vi "Impedance_Analyzer_Main.vi"() -> ()   [LabVIEW 2022 SP3]
uses:
  <vilib>/Math Plots/2D Math Plots/2D Compass/2D Compass XCtrl/2D Compass.xctl
  <vilib>/Math Plots/2D Math Plots/2D Compass/2D Compass Datatype/2D Compass Datatype.lvclass
  <vilib>/Analysis/1siggen.llb/Ramp Pattern by Samples.vi
  <vilib>/Analysis/baseanly.llb/Mean (DBL).vi
  <vilib>/Math Plots/2D Math Plots/2D Compass/2D Compass Datatype/Public/Plot Helper (Vector).vi
  <vilib>/Analysis/NI_AALBase.lvlib
panel:
  in  "Shunt Gain Setting 3":bool
  in  "ResetLine-Shunt 2":tag="PXI1Slot2/port0/line3"
  in  "SetLine-Shunt 2":tag="PXI1Slot2/port0/line2"
  in  "SetLine-Shunt":tag="PXI1Slot2/port0/line0"
  in  "ResetLine-Shunt":tag="PXI1Slot2/port0/line1"
  in  "Shunt Gain Setting":bool
  out "Test Number 3":i32=2
  in  "Saving Cluster":T1={"Experiment Title"="Experiment Title", "Save Path"=path "C:/Users/MPI/Downloads", "File Name String"="TestStats", "Meta-Data Array"=[]}
  out "Main loop has stopped":bool
  out "Duration of last non-idle state (sec)":dbl format="%.3g"
  out "Start of current operation":timestamp=timestamp(3746717327.8850594 s since 1904-01-01)
  out "Current system state":string="Idle"
  in  "stop":bool
  in  "Tab Control":T2(tab)
  in  "Test Params Cluster":T3={"Test Freq. (Hz)"=100.0, "Output Signal Amplitude\nVolts Pk"=0.6, "Sampling Time (s)"=0.1, "Sampling Rate (Hz)"=1000000.0, "Output Channel"="PXI1Slot2/ao0", "Current Channel"="PXI1Slot2/ai0", "Voltage Channel"="PXI1Slot2/ai1", "Trigger Channel"="/PXI1Slot2/ao/StartTrigger", "Number of runs"=5} {"Sampling Rate (Hz)" format="%#_6p"}
  in  "LCR Params":T4={"Rg_Vmon"=10000.0, "Rg_Imon"=10000.0, "ESL_Cal"=3.9470118585717184e-07, "ESR_Cal"=-0.006312489258536832, "Cp_Cal"=0.0, "Rp_Cal"=1000000000.0, "UseCorrection"=TRUE, "R_Shunt"=100.0, "RLoad"=1000000000.0, "RLoad_Meas"=1000000000.0} {"RLoad_Meas" format="%#_6p"; "RLoad" format="%#_6p"; "R_Shunt" format="%#_6p"; "Rg_Vmon" format="%#_6p"; "Rg_Imon" format="%#_6p"; "ESL_Cal" format="%#_6p"; "ESR_Cal" format="%#_6p"; "Cp_Cal" format="%#_6p"; "Rp_Cal" format="%#_6p"}
  out "mean Real(Z)":dbl=-0.006312489258536832
  in  "Open Comp":bool
  in  "Short Comp":bool
  in  "Number of Tests\n-Compensation":i32=10 format="%#.6p"
  in  "Save final stats - Compensation":bool
  out "Histogram Graph Phase 2":T5(graph)={"X Values"=[0.059615962899507886, 0.05963710991927518, 0.05965825693904247, 0.05967940395880976, 0.05970055097857705, 0.05972169799834434, 0.05974284501811163, 0.059763992037878924, 0.059785139057646215, 0.059806286077413506], "Histogram: h(x)"=[1, 0, 0, 0, 0, 0, 0, 0, 0, 1]}
  out "Histogram Graph Phase 3":T5(graph)={"X Values"=[95.20701436407293, 95.2415389303248, 95.27606349657665, 95.31058806282851, 95.34511262908038, 95.37963719533224, 95.4141617615841, 95.44868632783596, 95.48321089408782, 95.51773546033968], "Histogram: h(x)"=[1, 0, 0, 2, 1, 1, 2, 1, 1, 1]}
  out "Histogram Graph Mag 3":T5(graph)={"X Values"=[0.05657083132191394, 0.05658175212173795, 0.05659267292156196, 0.05660359372138597, 0.05661451452120998, 0.05662543532103399, 0.056636356120858, 0.05664727692068201, 0.05665819772050602, 0.056669118520330033], "Histogram: h(x)"=[1, 0, 1, 0, 1, 0, 4, 1, 1, 1]}
  out "Histogram Graph Mag 2":T5(graph)={"X Values"=[91.42562370503113, 92.47253112610193, 93.51943854717271, 94.5663459682435, 95.61325338931428, 96.66016081038507, 97.70706823145585, 98.75397565252663, 99.80088307359742, 100.8477904946682], "Histogram: h(x)"=[1, 0, 0, 0, 0, 0, 0, 0, 0, 1]}
  out "Open Comp Output":T6 {"Mean |Z|" format="%#_6p"; "standard deviation |Z|" format="%#_6p"; "Mean Phase" format="%#_6p"; "standard deviation Phase" format="%#_6p"; "mean Ls" format="%#_6p"; "Standard dev. Ls" format="%#_6p"; "mean Real(Z)" format="%#_6p"; "Std. dev Real(Z)" format="%#_6p"; "mean Cs" format="%#_6p"; "Std. Dev. Cs" format="%#_6p"; "Mean Rp" format="%#_6p"; "Std. Dev. Rp" format="%#_6p"; "Mean Cp" format="%#_6p"; "Std. Dev. Cp" format="%#_6p"}
  out "Short Comp Output":T6={"Mean |Z|"=0.05952615930946873, "standard deviation |Z|"=0.00033736666024453306, "Mean Phase"=96.11062136035359, "standard deviation Phase"=5.234732094839484, "mean Ls"=3.9470118585717184e-07, "Standard dev. Ls"=4.734939240935585e-09, "mean Real(Z)"=-0.006312489258536832, "Std. dev Real(Z)"=0.005405474422231036, "mean Cs"=-0.00011330769248196087, "Std. Dev. Cs"=1.3530545947492297e-06, "Mean Rp"=-1.5539543323796643, "Std. Dev. Rp"=1.9485966785903661, "Mean Cp"=-0.00011139347112511099, "Std. Dev. Cp"=1.2568699443711718e-06} {"Mean |Z|" format="%#_6p"; "standard deviation |Z|" format="%#_6p"; "Mean Phase" format="%#_6p"; "standard deviation Phase" format="%#_6p"; "mean Ls" format="%#_6p"; "Standard dev. Ls" format="%#_6p"; "mean Real(Z)" format="%#_6p"; "Std. dev Real(Z)" format="%#_6p"; "mean Cs" format="%#_6p"; "Std. Dev. Cs" format="%#_6p"; "Mean Rp" format="%#_6p"; "Std. Dev. Rp" format="%#_6p"; "Mean Cp" format="%#_6p"; "Std. Dev. Cp" format="%#_6p"}
  out "Ls Chart 3":dbl(graph)
  out "ESR 3":dbl(graph)
  out "Ls Chart 2":dbl(graph)=3.933790349340922e-07
  out "ESR Short":dbl(graph)=-0.00624352369104645
  out "Current Short Comp. Results":T7={"|Z|"=0.05915622895148479, "Phase(Z)"=96.05844988136137, "Re(Z)"=-0.00624352369104645, "Imag(Z)"=0.058825826264318884, "Ls"=3.933790349340922e-07, "Cs"=-0.00011367766349435693, "Rp"=-0.5604942972794196, "Cp"=-0.00011241137195737807} {"|Z|" format="%#_6p"; "Phase(Z)" format="%#_6p"; "Re(Z)" format="%#_6p"; "Imag(Z)" format="%#_6p"; "Ls" format="%#_6p"; "Cs" format="%#_6p"; "Rp" format="%#_6p"; "Cp" format="%#_6p"}
  out "Current Open Comp. Results":T7={"|Z|"=0.05656537092200194, "Phase(Z)"=95.45920483054104, "Re(Z)"=-0.005381459479146001, "Imag(Z)"=0.056308801100875626, "Ls"=3.584729613913086e-07, "Cs"=-0.00011305866221997783, "Rp"=-0.5945675517845621, "Cp"=-0.00011203536283595137} {"|Z|" format="%#_6p"; "Phase(Z)" format="%#_6p"; "Re(Z)" format="%#_6p"; "Imag(Z)" format="%#_6p"; "Ls" format="%#_6p"; "Cs" format="%#_6p"; "Rp" format="%#_6p"; "Cp" format="%#_6p"}
  in  "Update Variables":bool
  out "Progress 3":i32(slide)=66 scale=0.0..100.0
  in  "Samples\nShort Comp":i32=3 format="%#.6p"
  out "Debug Cluster-Short":T8={"detected fundamental frequency"=23800.1359424882, "THD-IMon"=0.04051349221415451, "THD-VMon"=0.0, "IMon-Ampl"=0.9038077003743037, "VMon-Ampl"=0.0007818146474553097} {"VMon-Ampl" format="%.2p"; "IMon-Ampl" format="%.2p"; "THD-VMon" format="%.2p"; "THD-IMon" format="%.2p"; "detected fundamental frequency" format="%.2p"}
  out "Debug Cluster-Open":T8 {"VMon-Ampl" format="%.2p"; "IMon-Ampl" format="%.2p"; "THD-VMon" format="%.2p"; "THD-IMon" format="%.2p"; "detected fundamental frequency" format="%.2p"}
  in  "Start Stats":bool
  in  "Save final stats":bool
  out "Histogram Graph Phase":T5(graph)={"X Values"=[100.0, 100.0, 100.0, 100.0, 100.0, 100.0, 100.0, 100.0, 100.0, 100.0], "Histogram: h(x)"=[0, 0, 0, 0, 0, 0, 0, 0, 0, 2]}
  out "Progress":i32(slide)=66 scale=0.0..100.0
  out "Inductance Chart":dbl(graph)=3.606768335066755e-19
  out "output cluster":T6={"Mean |Z|"=100.0, "standard deviation |Z|"=0.0, "Mean Phase"=179.99999999999997, "standard deviation Phase"=0.0, "mean Ls"=3.606768335066755e-19, "Standard dev. Ls"=0.0, "mean Real(Z)"=-100.0, "Std. dev Real(Z)"=0.0, "mean Cs"=-112367830.95520051, "Std. Dev. Cs"=1.8250120749944284e-08, "Mean Rp"=-100.0, "Std. Dev. Rp"=0.0, "Mean Cp"=-3.6067683350667554e-23, "Std. Dev. Cp"=0.0} {"Mean |Z|" format="%#_6p"; "standard deviation |Z|" format="%#_6p"; "Mean Phase" format="%#_6p"; "standard deviation Phase" format="%#_6p"; "mean Ls" format="%#_6p"; "Standard dev. Ls" format="%#_6p"; "mean Real(Z)" format="%#_6p"; "Std. dev Real(Z)" format="%#_6p"; "mean Cs" format="%#_6p"; "Std. Dev. Cs" format="%#_6p"; "Mean Rp" format="%#_6p"; "Std. Dev. Rp" format="%#_6p"; "Mean Cp" format="%#_6p"; "Std. Dev. Cp" format="%#_6p"}
  out "Current Run Results":T7={"|Z|"=100.0, "Phase(Z)"=179.99999999999997, "Re(Z)"=-100.0, "Imag(Z)"=5.6654984523230034e-14, "Ls"=3.606768335066755e-19, "Cs"=-112367830.95520052, "Rp"=-100.0, "Cp"=-3.6067683350667554e-23} {"|Z|" format="%#_6p"; "Phase(Z)" format="%#_6p"; "Re(Z)" format="%#_6p"; "Imag(Z)" format="%#_6p"; "Ls" format="%#_6p"; "Cs" format="%#_6p"; "Rp" format="%#_6p"; "Cp" format="%#_6p"}
  out "Capacitance Chart":dbl(graph)=-112367830.95520052
  out "Phase Chart":dbl(graph)=179.99999999999997
  out "Real(Z) Chart":dbl(graph)=-100.0
  out "|Z| over time":dbl(graph)=100.0
  out "Test Number":i32=2
  in  "samples":i32=3 format="%#.6p"
  in  "Save Every\nRun File?":bool
  out "Debug Cluster-Stats":T8 {"VMon-Ampl" format="%.2p"; "IMon-Ampl" format="%.2p"; "THD-VMon" format="%.2p"; "THD-IMon" format="%.2p"; "detected fundamental frequency" format="%.2p"}
  in  "Start Freq. Sweep":bool
  in  "Save sweep":bool
  out "Mag Phase Graph":cluster{dbl[], dbl[]}[](graph)=[{[15000.0, 15213.695804509916, 15430.43600214417, 15650.263964505297, 15873.22368108446, 16099.359768064103, 16328.717477246168, 16561.34270510718, 16797.28200198266, 17036.582581382234, 17279.292329437434, 17525.459814484173, 17775.134296781664, 18028.365738369826, 18285.204813067154, 18545.70291661091, 18809.91217694204, 19077.8854646362, 19349.67640348376, 19625.339381220358, 19904.929560410354, 20188.502889485353, 20476.11611393997, 20767.82678768709, 21063.69328457491, 21363.774810068015, 21668.13141309509, 21976.823998064945, 22289.914337054226, 22607.46508216848, 22929.539778079397, 23256.202874740644, 23587.519740284875, 23923.556674104446, 24264.38092011853, 24610.060680229126, 24960.665127969078, 25316.264422344004, 25676.9297218719, 26042.73319882256, 26413.748053659852, 26790.048529689782, 27171.709927917225, 27558.80862211431, 27951.42207410347, 28349.628849258188, 28753.50863222483, 29163.142242867896, 29578.611652443007, 30000.0], [99.99999999999999, 100.00000000000001, 100.0, 100.0, 100.00000000000001, 100.00000000000001, 100.0, 100.0, 100.0, 99.99999999999999, 100.0, 100.0, 99.99999999999999, 100.00000000000001, 100.0, 100.0, 99.99999999999999, 100.0, 100.00000000000001, 100.00000000000001, 100.00000000000001, 99.99999999999999, 100.0, 99.99999999999999, 100.00000000000001, 100.00000000000001, 100.00000000000001, 100.00000000000001, 100.0, 99.99999999999999, 99.99999999999997, 100.0, 100.0, 99.99999999999999, 100.0, 99.99999999999999, 100.0, 100.00000000000001, 99.99999999999999, 100.0, 100.0, 100.00000000000001, 100.0, 100.0, 100.00000000000001, 100.00000000000001, 100.0, 100.0, 100.0, 100.00000000000001]}, {[15000.0, 15213.695804509916, 15430.43600214417, 15650.263964505297, 15873.22368108446, 16099.359768064103, 16328.717477246168, 16561.34270510718, 16797.28200198266, 17036.582581382234, 17279.292329437434, 17525.459814484173, 17775.134296781664, 18028.365738369826, 18285.204813067154, 18545.70291661091, 18809.91217694204, 19077.8854646362, 19349.67640348376, 19625.339381220358, 19904.929560410354, 20188.502889485353, 20476.11611393997, 20767.82678768709, 21063.69328457491, 21363.774810068015, 21668.13141309509, 21976.823998064945, 22289.914337054226, 22607.46508216848, 22929.539778079397, 23256.202874740644, 23587.519740284875, 23923.556674104446, 24264.38092011853, 24610.060680229126, 24960.665127969078, 25316.264422344004, 25676.9297218719, 26042.73319882256, 26413.748053659852, 26790.048529689782, 27171.709927917225, 27558.80862211431, 27951.42207410347, 28349.628849258188, 28753.50863222483, 29163.142242867896, 29578.611652443007, 30000.0], [-180.0, -180.0, -180.0, -180.0, -179.99999999999997, -180.0, -180.0, 179.99999999999997, -180.0, -180.0, -179.99999999999997, -179.99999999999997, 180.0, 179.99999999999994, 180.0, -180.0, -180.0, -180.0, -180.0, -179.99999999999997, 180.0, -179.99999999999997, -180.0, 180.0, 179.99999999999997, 179.99999999999997, 180.0, 180.0, 179.99999999999997, 180.0, -180.0, -180.0, 180.0, -180.0, 180.0, 179.99999999999997, 180.0, 180.0, 179.99999999999997, 180.0, 180.0, 179.99999999999997, 179.99999999999997, -180.0, -180.0, 180.0, 180.0, -179.99999999999997, -180.0, -180.0]}]
  in  "Freq Sweep Info":T9={"type"=1, "Number of\nTest Freqs"=50, "Start Freq"=15000.0, "Stop Freq"=30000.0} {"Stop Freq" format="%#.4p"; "Start Freq" format="%#.4p"; "type" items=["Linear", "Logarithmic"]}
  out "Current Run Cluster Sweep":T3={"Test Freq. (Hz)"=30000.0, "Output Signal Amplitude\nVolts Pk"=0.1, "Sampling Time (s)"=0.001, "Sampling Rate (Hz)"=2000000.0, "Output Channel"="SimDev1/ao0", "Current Channel"="SimDev1/ai0", "Voltage Channel"="SimDev1/ai1", "Trigger Channel"="/SimDev1/ao/StartTrigger", "Number of runs"=3}
  out "Current Run Impedances":T7={"|Z|"=100.00000000000001, "Phase(Z)"=-180.0, "Re(Z)"=-100.00000000000001, "Imag(Z)"=-1.2246063538223774e-14, "Ls"=-6.496738485085797e-20, "Cs"=433213885.68422616, "Rp"=-100.00000000000001, "Cp"=6.496738485085795e-24} {"|Z|" format="%#_6p"; "Phase(Z)" format="%#_6p"; "Re(Z)" format="%#_6p"; "Imag(Z)" format="%#_6p"; "Ls" format="%#_6p"; "Cs" format="%#_6p"; "Rp" format="%#_6p"; "Cp" format="%#_6p"}
  out "RealImag Graph":cluster{dbl[], dbl[]}[](graph)=[{[15000.0, 15213.695804509916, 15430.43600214417, 15650.263964505297, 15873.22368108446, 16099.359768064103, 16328.717477246168, 16561.34270510718, 16797.28200198266, 17036.582581382234, 17279.292329437434, 17525.459814484173, 17775.134296781664, 18028.365738369826, 18285.204813067154, 18545.70291661091, 18809.91217694204, 19077.8854646362, 19349.67640348376, 19625.339381220358, 19904.929560410354, 20188.502889485353, 20476.11611393997, 20767.82678768709, 21063.69328457491, 21363.774810068015, 21668.13141309509, 21976.823998064945, 22289.914337054226, 22607.46508216848, 22929.539778079397, 23256.202874740644, 23587.519740284875, 23923.556674104446, 24264.38092011853, 24610.060680229126, 24960.665127969078, 25316.264422344004, 25676.9297218719, 26042.73319882256, 26413.748053659852, 26790.048529689782, 27171.709927917225, 27558.80862211431, 27951.42207410347, 28349.628849258188, 28753.50863222483, 29163.142242867896, 29578.611652443007, 30000.0], [-99.99999999999999, -100.00000000000001, -100.0, -100.0, -100.00000000000001, -100.00000000000001, -100.0, -100.0, -100.0, -99.99999999999999, -100.0, -100.0, -99.99999999999999, -100.00000000000001, -100.0, -100.0, -99.99999999999999, -100.0, -100.00000000000001, -100.00000000000001, -100.00000000000001, -99.99999999999999, -100.0, -99.99999999999999, -100.00000000000001, -100.00000000000001, -100.00000000000001, -100.00000000000001, -100.0, -99.99999999999999, -99.99999999999997, -100.0, -100.0, -99.99999999999999, -100.0, -99.99999999999999, -100.0, -100.00000000000001, -99.99999999999999, -100.0, -100.0, -100.00000000000001, -100.0, -100.0, -100.00000000000001, -100.00000000000001, -100.0, -100.0, -100.0, -100.00000000000001]}, {[15000.0, 15213.695804509916, 15430.43600214417, 15650.263964505297, 15873.22368108446, 16099.359768064103, 16328.717477246168, 16561.34270510718, 16797.28200198266, 17036.582581382234, 17279.292329437434, 17525.459814484173, 17775.134296781664, 18028.365738369826, 18285.204813067154, 18545.70291661091, 18809.91217694204, 19077.8854646362, 19349.67640348376, 19625.339381220358, 19904.929560410354, 20188.502889485353, 20476.11611393997, 20767.82678768709, 21063.69328457491, 21363.774810068015, 21668.13141309509, 21976.823998064945, 22289.914337054226, 22607.46508216848, 22929.539778079397, 23256.202874740644, 23587.519740284875, 23923.556674104446, 24264.38092011853, 24610.060680229126, 24960.665127969078, 25316.264422344004, 25676.9297218719, 26042.73319882256, 26413.748053659852, 26790.048529689782, 27171.709927917225, 27558.80862211431, 27951.42207410347, 28349.628849258188, 28753.50863222483, 29163.142242867896, 29578.611652443007, 30000.0], [1.2246063538223771e-14, 1.2246063538223774e-14, 1.2246063538223773e-14, 1.2246063538223773e-14, 5.665498452323004e-14, 1.2246063538223774e-14, 1.2246063538223773e-14, 5.6654984523230034e-14, 1.2246063538223773e-14, 1.2246063538223771e-14, 5.6654984523230034e-14, 5.6654984523230034e-14, 1.2246063538223771e-14, 1.0106390550823631e-13, 1.2246063538223773e-14, 1.2246063538223773e-14, 1.2246063538223771e-14, 1.2246063538223773e-14, 1.2246063538223774e-14, 5.665498452323004e-14, 1.2246063538223774e-14, 5.665498452323003e-14, 1.2246063538223773e-14, 1.2246063538223771e-14, 5.665498452323004e-14, 5.665498452323004e-14, 1.2246063538223774e-14, 1.2246063538223774e-14, 5.6654984523230034e-14, 1.2246063538223771e-14, 1.224606353822377e-14, 1.2246063538223773e-14, 1.2246063538223773e-14, 1.2246063538223771e-14, 1.2246063538223773e-14, 5.665498452323003e-14, 1.2246063538223773e-14, 1.2246063538223774e-14, 5.665498452323003e-14, 1.2246063538223773e-14, 1.2246063538223773e-14, 5.665498452323004e-14, 5.6654984523230034e-14, 1.2246063538223773e-14, 1.2246063538223774e-14, 1.2246063538223774e-14, 1.2246063538223773e-14, 5.6654984523230034e-14, 1.2246063538223773e-14, 1.2246063538223774e-14]}]
  out "Mean Mag":dbl=100.0 format="%.4p"
  out "Mean Phase":dbl=-7.2 format="%0.2f"
  out "Progress 2":i32(slide)=98 scale=0.0..100.0
  out "Test Number 2":i32=49
  out "Impedance Vector":refnum<class "2D Plot Datatype.lvclass">[](xcontrol) caption="2D Compass"
  out "Progress Single Run":i32(slide)=66 scale=0.0..100.0
  in  "Start Single Meas":bool
  in  "Save Single Impedance":bool
  out "Mean Signal\nImpedance cluster":T7={"|Z|"=0.007576457903951982, "Phase(Z)"=5.046854007613568, "Re(Z)"=0.0075470846798780635, "Imag(Z)"=0.0006665037172486679, "Ls"=4.457031982741531e-09, "Cs"=-0.01003322608680636, "Rp"=0.007605945448499181, "Cp"=-7.764496908604732e-05} {"|Z|" format="%#_6p"; "Phase(Z)" format="%#_6p"; "Re(Z)" format="%#_6p"; "Imag(Z)" format="%#_6p"; "Ls" format="%#_6p"; "Cs" format="%#_6p"; "Rp" format="%#_6p"; "Cp" format="%#_6p"}
  out "Debug Cluster-Single":T8={"detected fundamental frequency"=23800.0328131461, "THD-IMon"=0.040850349277074975, "THD-VMon"=0.0, "IMon-Ampl"=0.7425195895412117, "VMon-Ampl"=0.0037497807912680457} {"VMon-Ampl" format="%.2p"; "IMon-Ampl" format="%.2p"; "THD-VMon" format="%.2p"; "THD-IMon" format="%.2p"; "detected fundamental frequency" format="%.2p"}
  # "Open Impedance Analyzer"
  # "TODO ensure sampling time isn't below one period"
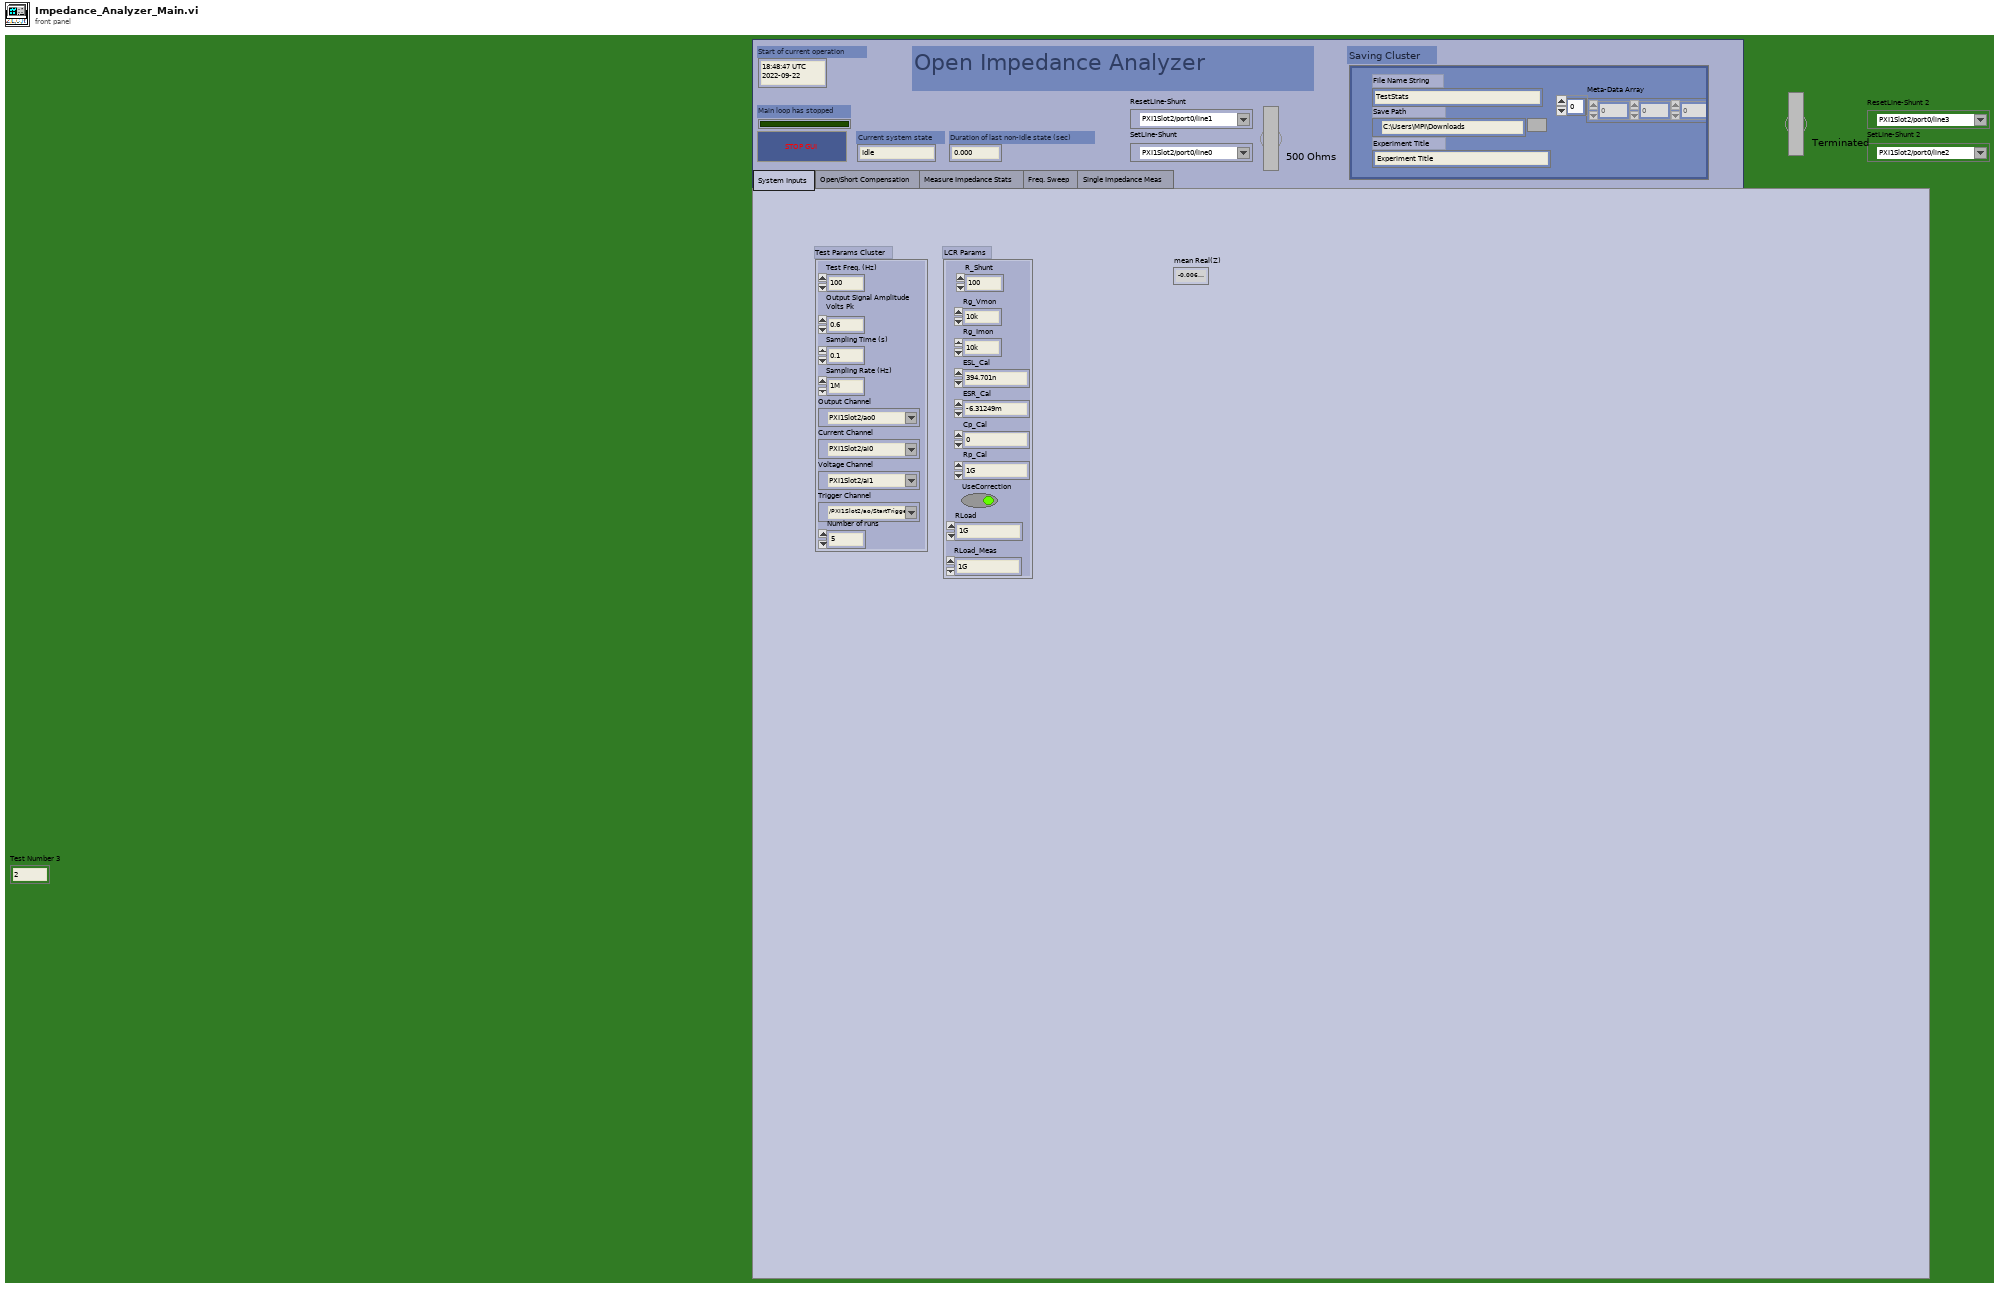
[diagram p1: front panel]
types:
  T1 = cluster{"Experiment Title":string, "Save Path":path, "File Name String":string, "Meta-Data Array":dbl[]}
  T2 = enum32{"System Inputs", "Open/Short Compensation", "Measure Impedance Stats", "Freq. Sweep", "Single Impedance Meas"}
  T3 = cluster{"Test Freq. (Hz)":dbl, "Output Signal Amplitude\nVolts Pk":dbl, "Sampling Time (s)":dbl, "Sampling Rate (Hz)":dbl, "Output Channel":tag, "Current Channel":tag, "Voltage Channel":tag, "Trigger Channel":tag, "Number of runs":i32}
  T4 = cluster{"Rg_Vmon":dbl, "Rg_Imon":dbl, "ESL_Cal":dbl, "ESR_Cal":dbl, "Cp_Cal":dbl, "Rp_Cal":dbl, "UseCorrection":bool, "R_Shunt":dbl, "RLoad":dbl, "RLoad_Meas":dbl}
  T5 = cluster{"X Values":dbl[], "Histogram: h(x)":i32[]}
  T6 = cluster{"Mean |Z|":dbl, "standard deviation |Z|":dbl, "Mean Phase":dbl, "standard deviation Phase":dbl, "mean Ls":dbl, "Standard dev. Ls":dbl, "mean Real(Z)":dbl, "Std. dev Real(Z)":dbl, "mean Cs":dbl, "Std. Dev. Cs":dbl, "Mean Rp":dbl, "Std. Dev. Rp":dbl, "Mean Cp":dbl, "Std. Dev. Cp":dbl}
  T7 = cluster{"|Z|":dbl, "Phase(Z)":dbl, "Re(Z)":dbl, "Imag(Z)":dbl, "Ls":dbl, "Cs":dbl, "Rp":dbl, "Cp":dbl}
  T8 = cluster{"detected fundamental frequency":dbl, "THD-IMon":dbl, "THD-VMon":dbl, "IMon-Ampl":dbl, "VMon-Ampl":dbl}
  T9 = cluster{"type":u16, "Number of\nTest Freqs":i32, "Start Freq":dbl, "Stop Freq":dbl}
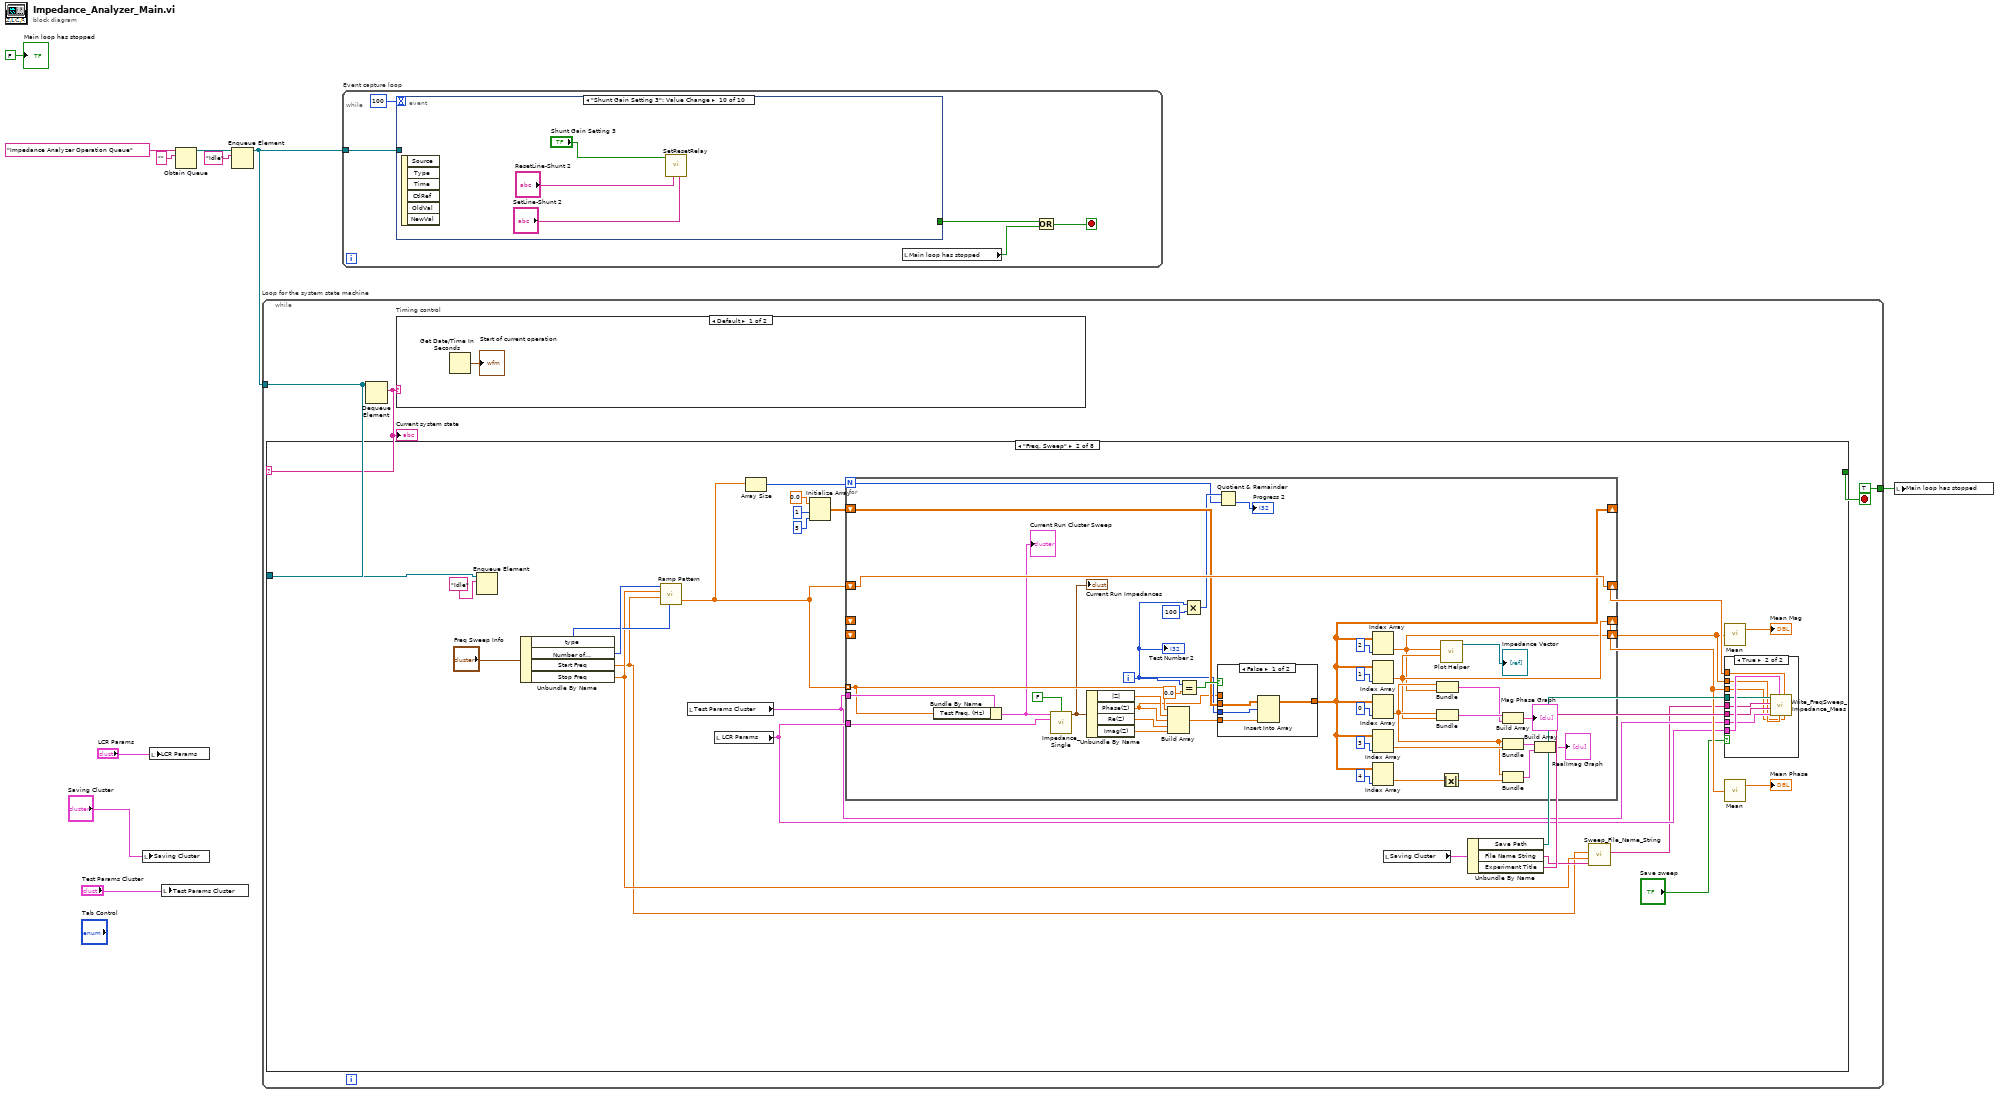
[diagram p0: block diagram]
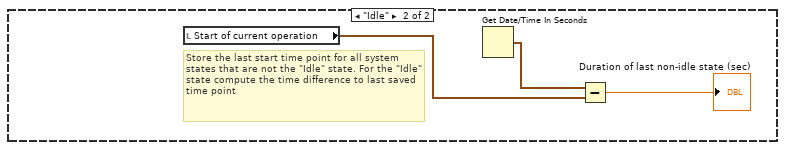
[diagram p2: hidden frame]
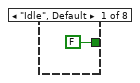
[diagram p3: hidden frame]
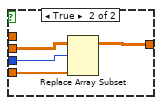
[diagram p5: hidden frame]
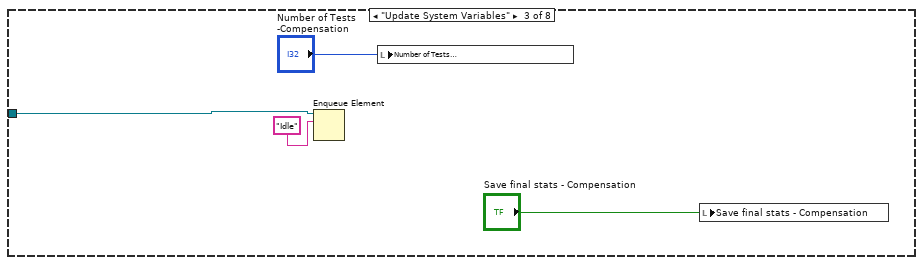
[diagram p6: hidden frame]
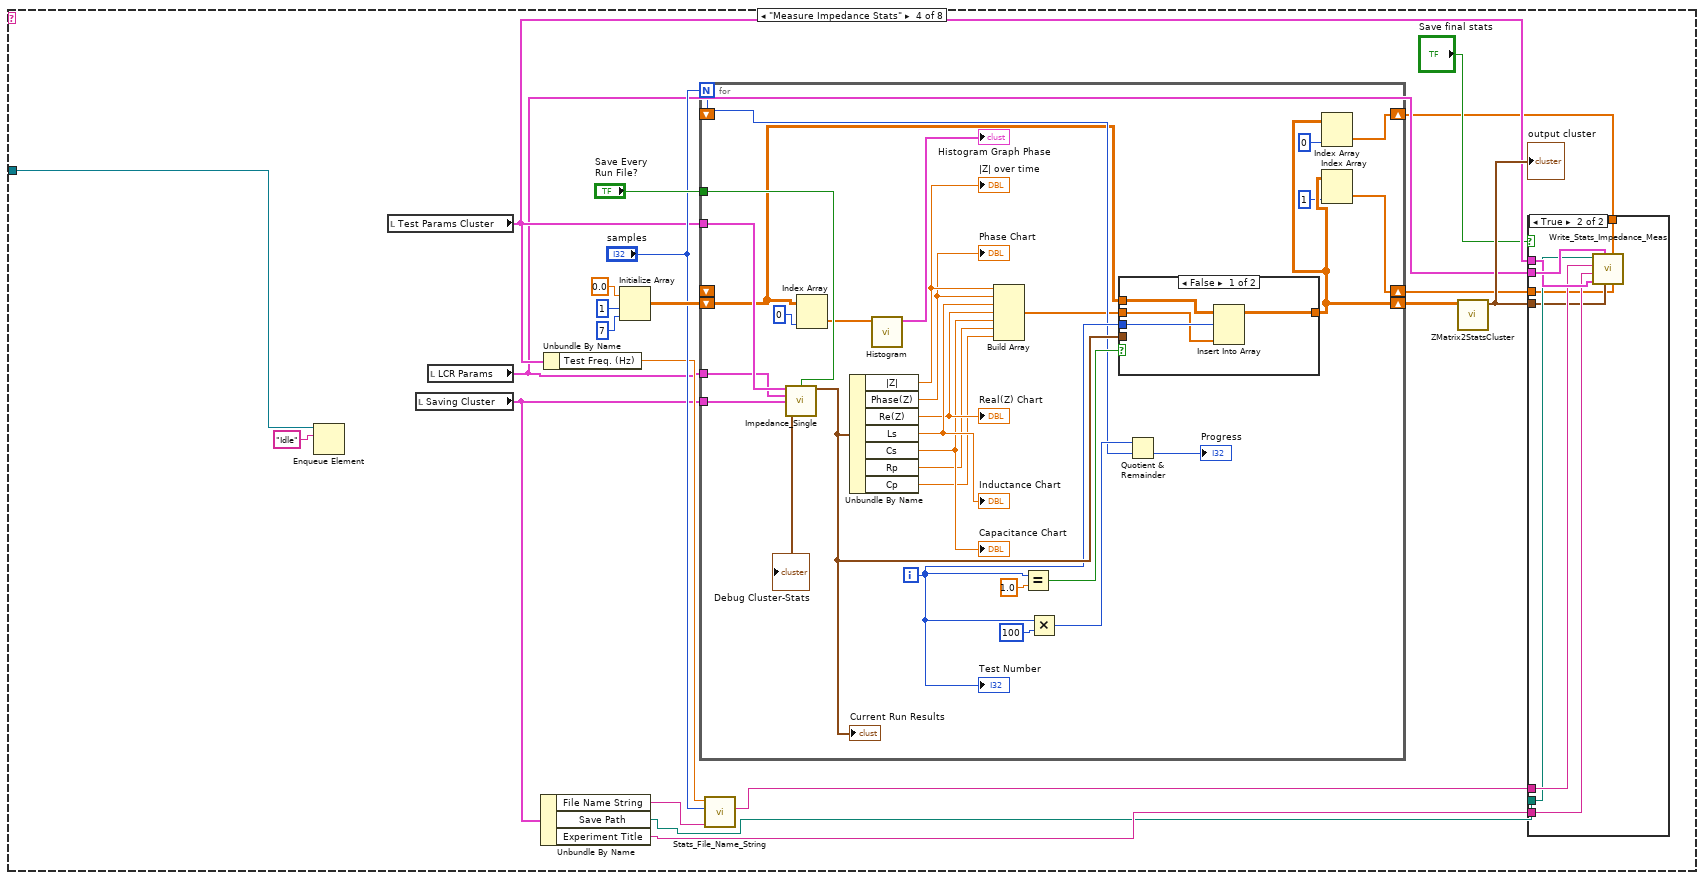
[diagram p7: hidden frame]
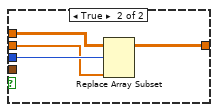
[diagram p8: hidden frame]
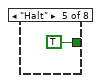
[diagram p10: hidden frame]
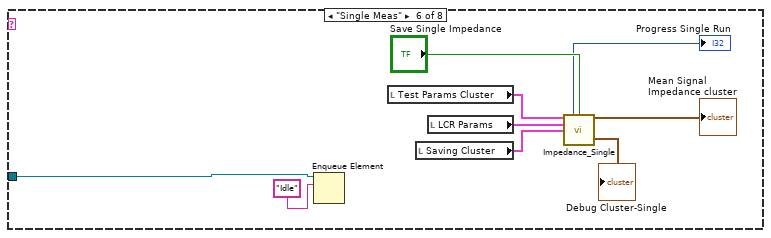
[diagram p11: hidden frame]
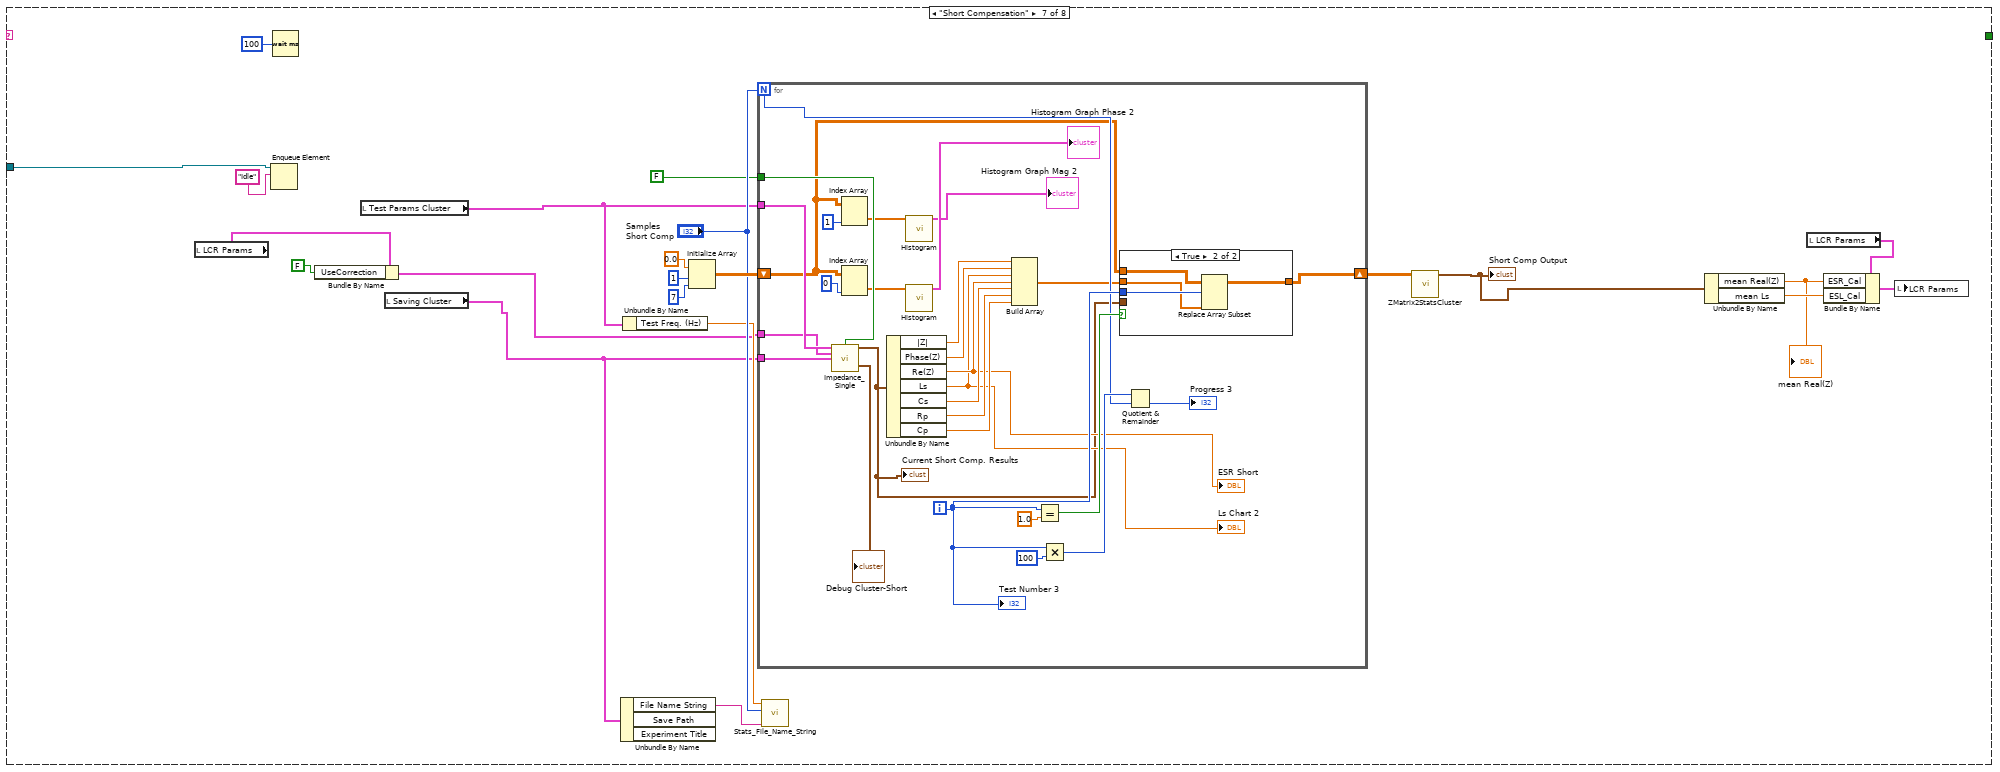
[diagram p12: hidden frame]
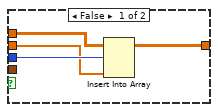
[diagram p13: hidden frame]
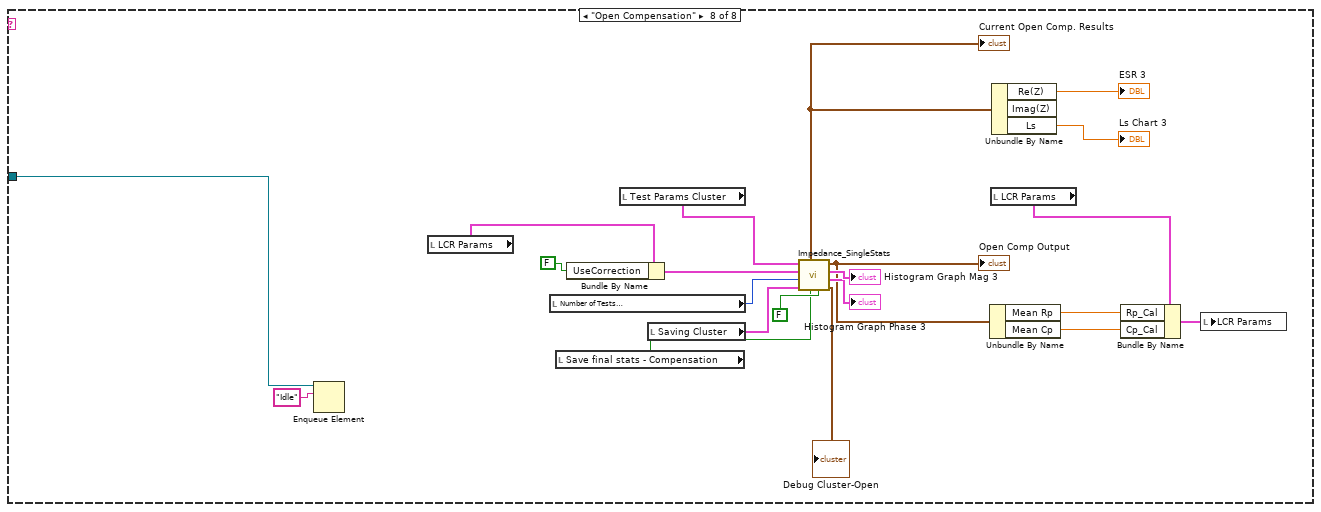
[diagram p14: hidden frame]
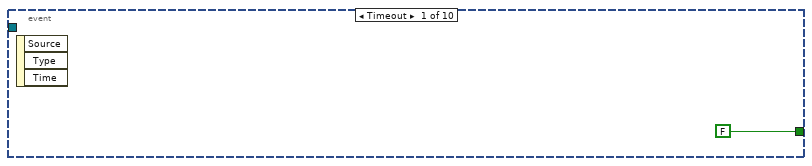
[diagram p15: hidden frame]
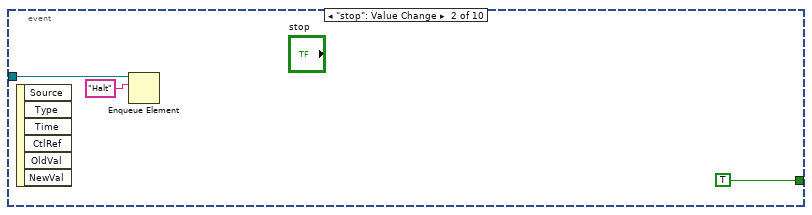
[diagram p16: hidden frame]
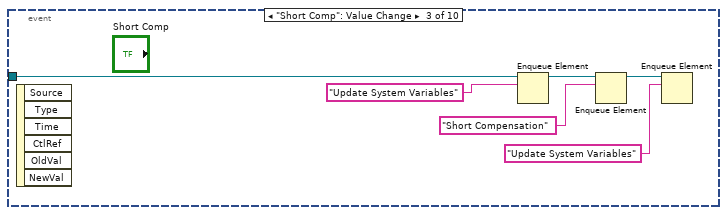
[diagram p17: hidden frame]
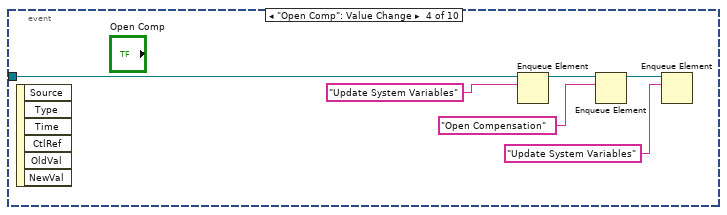
[diagram p18: hidden frame]
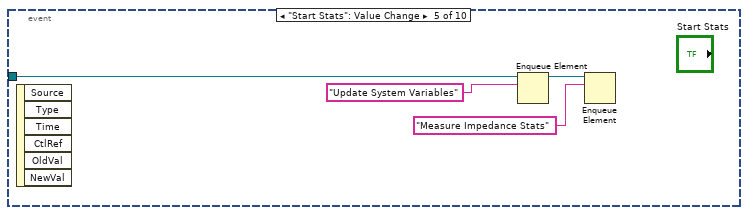
[diagram p19: hidden frame]
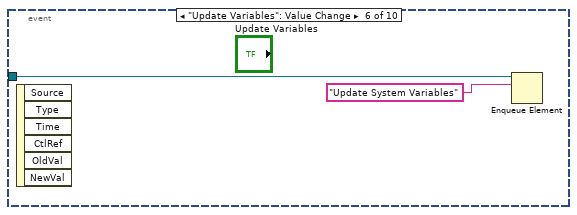
[diagram p20: hidden frame]
diagram:
  n1 = local write "Saving Cluster"("Saving Cluster") -> ()
  n2 = local write "LCR Params"("LCR Params") -> ()
  n3 = local write "Test Params Cluster"("Test Params Cluster") -> ()
  n4 = Obtain Queue(name (unnamed)="Impedance Analyzer Operation Queue", element data type="" ("Type def")) -> (queue out=w7:refnum<queue>)  [unwired: 3 in, 2 out]
  n5 = Enqueue Element(queue=w7, element="Idle") -> (queue out=w5:refnum<queue>)  [unwired: 2 in, 2 out]
  n6 = while "Loop for the system state machine" {
    tunnel: w5 -> [w13]
    tunnel: [TRUE ("Main loop has stopped")] -> w1
    stop <- w14 stop-if-true
    n7 = Dequeue Element(queue=w13) -> (element=w12:string)  [unwired: 2 in, 3 out]
    "Current system state" <- w12
    n8 = case shown="\"Freq. Sweep\"" w12 {
      tunnel: [FALSE _ _ _ TRUE _ _ _] -> w14
      tunnel: w13 -> [_ w45 w103 w124 _ w174 w198 w242]
      frame "Idle", Default {
      }
      frame "Freq. Sweep" {
        n9 = Enqueue Element(queue=w45, element="Idle") -> ()  [unwired: 2 in, 3 out]
        n10 = Unbundle By Name("Freq Sweep Info") -> ("type"=w32:u16, "Number of\nTest Freqs"=w33:i32, "Start Freq"=w20:dbl, "Stop Freq"=w21:dbl)
        n11 = call-poly <vilib>:"Ramp Pattern.vi"("type"=w32, "start"=w20, "end"=w21, "samples"=w33) -> ("Ramp Pattern"=w39:dbl[])  [unwired: 6 in, 1 out]
        n12 = local read "Test Params Cluster"() -> (w25:T3)
        n13 = local read "LCR Params"() -> (w26:T4)
        n14 = Array Size(array=w39) -> (size(s)=w43:i32)
        n15 = Initialize Array(0.0 ("element"), 1 ("dimension size"), 5 ("dimension size")) -> (w36:dbl[][])
        n16 = for {
          N: w43 -> [w78]
          shift-right: [w87] -> w40
          shift-left: w39 -> [w87]
          tunnel: w25 -> [w88]
          tunnel: w26 -> [w92]
          tunnel: w39 -> [w76] mode=indexing
          shift-right: [w58] -> _
          shift-left: w36 -> [w86]
          shift-right: [w60] -> w30
          shift-left: _ -> [_]
          shift-right: [w59] -> w29
          shift-left: _ -> [_]
          i -> [w77]
          n17 = Bundle By Name(cluster=w88, "Test Freq. (Hz)"=w76) -> (w57:T3)
          "Current Run Cluster Sweep" <- w57
          n18 = call "Impedance_Single.vi"("Test Params Cluster"=w57, "SaveFile?"=FALSE, "LCR Params"=w92) -> ("Mean Signal\nImpedance cluster"=w54:T7)  [unwired: 10 in, 2 out]
          "Current Run Impedances" <- w54
          n19 = Unbundle By Name(w54) -> ("|Z|"=w75:dbl, "Phase(Z)"=w74:dbl, "Re(Z)"=w73:dbl, "Imag(Z)"=w72:dbl)
          n20 = Build Array(w76, w75, w74, w73, w72) -> (w71:dbl[])
          n21 = Equal?(x=w77, y=0.0) -> (x = y?=w89:bool)
          n22 = Multiply(x=w77, y=100) -> (x*y=w79:i32)
          n23 = case shown="False" w89 {
            tunnel: [w93 w100] -> w58
            tunnel: w74 -> [_ _]
            tunnel: w77 -> [w96 w99]
            tunnel: w86 -> [w95 w98]
            tunnel: w71 -> [w94 w97]
            frame False {
              n24 = Insert Into Array(array=w95, index (row)=w96, new element=w94) -> (w93:dbl[][])  [unwired: 1 in]
            }
            frame True {
              n25 = Replace Array Subset(array=w98, new element=w97, index (row)=w99) -> (w100:dbl[][])  [unwired: 1 in]
            }
          }
          n26 = Quotient & Remainder(x=w79, y=w78) -> (floor(x/y)=→"Progress 2":i32)  [unwired: 1 out]
          n27 = Index Array(array=w58, index (col)=2 ("disabled index (col)")) -> (element=w59:dbl[])  [unwired: 1 in]
          n28 = Index Array(array=w58, index (col)=1 ("disabled index (col)")) -> (element=w60:dbl[])  [unwired: 1 in]
          n29 = Index Array(array=w58, index (col)=0 ("disabled index (col)")) -> (element=w63:dbl[])  [unwired: 1 in]
          n30 = Index Array(array=w58, index (col)=3 ("disabled index (col)")) -> (element=w64:dbl[])  [unwired: 1 in]
          n31 = Index Array(array=w58, index (col)=4 ("disabled index (col)")) -> (element=w65:dbl[])  [unwired: 1 in]
          n32 = Bundle(w63, w59) -> (w61:cluster{dbl[], dbl[]})  [unwired: 1 in]
          n33 = Bundle(w63, w60) -> (w84:cluster{dbl[], dbl[]})  [unwired: 1 in]
          n34 = Absolute Value(x=w65) -> (abs(x)=w82:dbl[])
          n35 = call-poly <vilib>:"Plot Helper.vi"("radius vector"=w60, "theta vector"=w59) -> ("2D Plot Class Obj Array out"=→"Impedance Vector":refnum<class "2D Plot Datatype.lvclass">[])  [unwired: 2 in, 7 out]
          n36 = Build Array(w84, w61) -> (→"Mag Phase Graph":cluster{dbl[], dbl[]}[])
          n37 = Bundle(w63, w64) -> (w62:cluster{dbl[], dbl[]})  [unwired: 1 in]
          n38 = Bundle(w63, w82) -> (w83:cluster{dbl[], dbl[]})  [unwired: 1 in]
          n39 = Build Array(w62, w83) -> (→"RealImag Graph":cluster{dbl[], dbl[]}[])
          "Test Number 2" <- w77
        }
        n40 = local read "Saving Cluster"() -> (w27:T1)
        n41 = Unbundle By Name(w27) -> ("Save Path"=w35:path, "File Name String"=w23:string, "Experiment Title"=w34:string)
        n42 = call "Sweep_File_Name_String.vi"("String"=w23, "Stop"=w21, "Start"=w20) -> ("Output string"=w22:string)  [unwired: 8 in]
        n43 = call-poly <vilib>:"Mean.vi"("X"=w30) -> ("mean"=→"Mean Mag":dbl)  [unwired: 1 out]
        n44 = case shown="True" "Save sweep" {
          tunnel: w26 -> [_ w53]
          tunnel: w35 -> [_ w52]
          tunnel: w22 -> [_ w51]
          tunnel: w34 -> [_ w50]
          tunnel: w25 -> [_ w49]
          tunnel: w40 -> [_ w48]
          tunnel: w30 -> [_ w47]
          tunnel: w29 -> [_ w46]
          frame False {
          }
          frame True {
            n45 = call "Write_FreqSweep_Impedance_Meas.vi"("Z_Phase_Vec"=w46, "Freq Vector"=w48, "|Z| Vector"=w47, "Compensation and Gain"=w53, "Test Params Cluster"=w49, "Experiment Title"=w50, "File Name String"=w51, "Path"=w52) -> ()  [unwired: 4 in]
          }
        }
        n46 = call-poly <vilib>:"Mean.vi"("X"=w29) -> ("mean"=→"Mean Phase":dbl)  [unwired: 1 out]
      }
      frame "Update System Variables" {
        n47 = Enqueue Element(queue=w103, element="Idle") -> ()  [unwired: 2 in, 3 out]
        n48 = local write "Number of Tests\n-Compensation"("Number of Tests\n-Compensation") -> ()
        n49 = local write "Save final stats - Compensation"("Save final stats - Compensation") -> ()
      }
      frame "Measure Impedance Stats" {
        n50 = Enqueue Element(queue=w124, element="Idle") -> ()  [unwired: 2 in, 3 out]
        n51 = local read "Test Params Cluster"() -> (w110:T3)
        n52 = local read "Saving Cluster"() -> (w109:T1)
        n53 = local read "LCR Params"() -> (w108:T4)
        n54 = Unbundle By Name(w109) -> ("File Name String"=w117:string, "Save Path"=w118:path, "Experiment Title"=w119:string)
        n55 = Unbundle By Name(w110) -> ("Test Freq. (Hz)"=w115:dbl)
        n56 = Initialize Array(0.0 ("element"), 1 ("dimension size"), 7 ("dimension size")) -> (w122:dbl[][])
        n57 = for {
          N: "samples" -> [w144]
          shift-right: [w131] -> w112
          shift-left: w122 -> [w134]
          tunnel: w110 -> [w152]
          tunnel: w108 -> [w151]
          tunnel: "Save Every\nRun File?" -> [w150]
          tunnel: w109 -> [w143]
          shift-right: [w128] -> w106
          shift-left: _ -> [_]
          shift-right: [w127] -> w105
          shift-left: _ -> [_]
          i -> [w145]
          n58 = call "Impedance_Single.vi"("Test Params Cluster"=w152, "SaveFile?"=w150, "LCR Params"=w151, "Saving Cluster"=w143) -> ("Mean Signal\nImpedance cluster"=w149:T7, "Debug Cluster"=→"Debug Cluster-Stats":T8)  [unwired: 9 in, 1 out]
          "Current Run Results" <- w149
          n59 = Index Array(array=w134, index (col)=0 ("disabled index (col)")) -> (element=w132:dbl[])  [unwired: 1 in]
          n60 = Unbundle By Name(w149) -> ("|Z|"=w142:dbl, "Phase(Z)"=w141:dbl, "Re(Z)"=w139:dbl, "Ls"=w140:dbl, "Cs"=w138:dbl, "Rp"=w137:dbl, "Cp"=w136:dbl)
          "|Z| over time" <- w142
          "Real(Z) Chart" <- w139
          "Phase Chart" <- w141
          "Inductance Chart" <- w140
          "Capacitance Chart" <- w138
          n61 = call <vilib>:"Histogram.vi"("X"=w132) -> ("Histogram Graph"=→"Histogram Graph Phase":T5)  [unwired: 7 in, 3 out]
          n62 = Build Array(w142, w141, w140, w139, w138, w137, w136) -> (w135:dbl[])
          n63 = Equal?(x=w145, y=1.0) -> (x = y?=w153:bool)
          n64 = Multiply(x=w145, y=100) -> (x*y=w146:i32)
          n65 = case shown="False" w153 {
            tunnel: w134 -> [w159 w163]
            tunnel: w145 -> [w157 w161]
            tunnel: [w158 w162] -> w131
            tunnel: w149 -> [_ _]
            tunnel: w135 -> [w156 w160]
            frame False {
              n66 = Insert Into Array(array=w159, index (row)=w157, new element=w156) -> (w158:dbl[][])  [unwired: 1 in]
            }
            frame True {
              n67 = Replace Array Subset(array=w163, new element=w160, index (row)=w161) -> (w162:dbl[][])  [unwired: 1 in]
            }
          }
          n68 = Quotient & Remainder(x=w146, y=w144) -> (floor(x/y)=→"Progress":i32)  [unwired: 1 out]
          n69 = Index Array(array=w131, index (col)=0 ("disabled index (col)")) -> (element=w128:dbl[])  [unwired: 1 in]
          n70 = Index Array(array=w131, index (col)=1 ("disabled index (col)")) -> (element=w127:dbl[])  [unwired: 1 in]
          "Test Number" <- w145
        }
        n71 = call "Stats_File_Name_String.vi"("String"=w117, "N"="samples", "TestFreq"=w115) -> ("Output string"=w114:string)  [unwired: 8 in]
        n72 = call "ZMatrix2StatsCluster.vi"("Array"=w112) -> ("output cluster 2"=w111:T6)  [unwired: 10 in]
        "output cluster" <- w111
        n73 = case shown="True" "Save final stats" {
          tunnel: w108 -> [_ w171]
          tunnel: w110 -> [_ w170]
          tunnel: w119 -> [_ w169]
          tunnel: w114 -> [_ w168]
          tunnel: w118 -> [_ w167]
          tunnel: w111 -> [_ w166]
          tunnel: w106 -> [_ w165]
          tunnel: w105 -> [_ w164]
          frame False {
          }
          frame True {
            n74 = call "Write_Stats_Impedance_Meas.vi"("Z Phase"=w164, "|Z| Mag"=w165, "Output Stats Cluster"=w166, "Compensation and Gain"=w171, "Test Params Cluster"=w170, "Experiment Title"=w169, "File Name String"=w168, "Path"=w167) -> ()  [unwired: 4 in]
          }
        }
      }
      frame "Halt" {
      }
      frame "Single Meas" {
        n75 = Enqueue Element(queue=w174, element="Idle") -> ()  [unwired: 2 in, 3 out]
        n76 = local read "Test Params Cluster"() -> (w181:T3)
        n77 = local read "Saving Cluster"() -> (w179:T1)
        n78 = local read "LCR Params"() -> (w180:T4)
        n79 = call "Impedance_Single.vi"("Test Params Cluster"=w181, "SaveFile?"="Save Single Impedance", "LCR Params"=w180, "Saving Cluster"=w179) -> ("Progress"=→"Progress Single Run":i32, "Mean Signal\nImpedance cluster"=→"Mean Signal\nImpedance cluster":T7, "Debug Cluster"=→"Debug Cluster-Single":T8)  [unwired: 9 in]
      }
      frame "Short Compensation" {
        n80 = local read "LCR Params"() -> (w200:T4)
        n81 = Enqueue Element(queue=w198, element="Idle") -> ()  [unwired: 2 in, 3 out]
        n82 = Wait (ms)(milliseconds to wait=u32 100) -> ()  [unwired: 1 out]
        n83 = Bundle By Name(cluster=w200, "UseCorrection"=FALSE) -> (w187:T4)
        n84 = local read "Test Params Cluster"() -> (w188:T3)
        n85 = local read "Saving Cluster"() -> (w186:T1)
        n86 = Unbundle By Name(w186) -> ("File Name String"=w193:string)  [unwired: 2 out]
        n87 = Unbundle By Name(w188) -> ("Test Freq. (Hz)"=w191:dbl)
        n88 = Initialize Array(0.0 ("element"), 1 ("dimension size"), 7 ("dimension size")) -> (w195:dbl[][])
        n89 = for {
          N: "Samples\nShort Comp" -> [w223]
          shift-right: [w213] -> w189
          shift-left: w195 -> [w206]
          tunnel: w188 -> [w230]
          tunnel: w187 -> [w229]
          tunnel: FALSE ("Save Every\nRun File?") -> [w228]
          tunnel: w186 -> [w222]
          i -> [w224]
          n90 = call "Impedance_Single.vi"("Test Params Cluster"=w230, "SaveFile?"=w228, "LCR Params"=w229, "Saving Cluster"=w222) -> ("Mean Signal\nImpedance cluster"=w209:T7, "Debug Cluster"=→"Debug Cluster-Short":T8)  [unwired: 9 in, 1 out]
          "Current Short Comp. Results" <- w209
          n91 = Index Array(array=w206, index (col)=1) -> (element=w207:dbl[])  [unwired: 1 in]
          n92 = Index Array(array=w206, index (col)=0 ("disabled index (col)")) -> (element=w214:dbl[])  [unwired: 1 in]
          n93 = Unbundle By Name(w209) -> ("|Z|"=w221:dbl, "Phase(Z)"=w220:dbl, "Re(Z)"=w211:dbl, "Ls"=w210:dbl, "Cs"=w219:dbl, "Rp"=w218:dbl, "Cp"=w217:dbl)
          "Ls Chart 2" <- w210
          "ESR Short" <- w211
          n94 = call <vilib>:"Histogram.vi"("X"=w207) -> ("Histogram Graph"=→"Histogram Graph Mag 2":T5)  [unwired: 7 in, 3 out]
          n95 = call <vilib>:"Histogram.vi"("X"=w214) -> ("Histogram Graph"=→"Histogram Graph Phase 2":T5)  [unwired: 7 in, 3 out]
          n96 = Build Array(w221, w220, w210, w211, w219, w218, w217) -> (w216:dbl[])
          n97 = Equal?(x=w224, y=1.0) -> (x = y?=w231:bool)
          n98 = Multiply(x=w224, y=100) -> (x*y=w225:i32)
          n99 = case shown="True" w231 {
            tunnel: w206 -> [w236 w240]
            tunnel: w224 -> [w234 w238]
            tunnel: [w235 w239] -> w213
            tunnel: w209 -> [_ _]
            tunnel: w216 -> [w233 w237]
            frame False {
              n100 = Insert Into Array(array=w236, index (row)=w234, new element=w233) -> (w235:dbl[][])  [unwired: 1 in]
            }
            frame True {
              n101 = Replace Array Subset(array=w240, new element=w237, index (row)=w238) -> (w239:dbl[][])  [unwired: 1 in]
            }
          }
          n102 = Quotient & Remainder(x=w225, y=w223) -> (floor(x/y)=→"Progress 3":i32)  [unwired: 1 out]
          "Test Number 3" <- w224
        }
        n103 = call "Stats_File_Name_String.vi"("String"=w193, "N"="Samples\nShort Comp", "TestFreq"=w191) -> ()  [unwired: 8 in, 1 out]
        n104 = call "ZMatrix2StatsCluster.vi"("Array"=w189) -> ("output cluster 2"=w184:T6)  [unwired: 10 in]
        "Short Comp Output" <- w184
        n105 = Unbundle By Name(w184) -> ("mean Real(Z)"=w182:dbl, "mean Ls"=w183:dbl)
        "mean Real(Z)" <- w182
        n106 = local read "LCR Params"() -> (w203:T4)
        n107 = Bundle By Name(cluster=w203, "ESR_Cal"=w182, "ESL_Cal"=w183) -> (w202:T4)
        n108 = local write "LCR Params"(w202) -> ()
      }
      frame "Open Compensation" {
        n109 = Enqueue Element(queue=w242, element="Idle") -> ()  [unwired: 2 in, 3 out]
        n110 = local read "LCR Params"() -> (w247:T4)
        n111 = local read "Number of Tests\n-Compensation"() -> (w244:i32)
        n112 = local read "Save final stats - Compensation"() -> (w245:bool)
        n113 = Bundle By Name(cluster=w247, "UseCorrection"=FALSE) -> (w248:T4)
        n114 = local read "Test Params Cluster"() -> (w259:T3)
        n115 = local read "Saving Cluster"() -> (w258:T1)
        n116 = call "Impedance_SingleStats.vi"("Save Every\nRun File?"=FALSE ("Save Every\nRun File?"), "Save final stats"=w245, "Saving Cluster"=w258, "samples"=w244, "LCR Params"=w248, "Test Params Cluster"=w259) -> ("Debug Cluster"=→"Debug Cluster-Open":T8, "Histogram Graph Phase"=→"Histogram Graph Phase 3":T5, "Histogram Graph Mag"=→"Histogram Graph Mag 3":T5, "output cluster"=w253:T6, "Current Run Results"=w257:T7)  [unwired: 1 out]
        "Open Comp Output" <- w253
        "Current Open Comp. Results" <- w257
        n117 = Unbundle By Name(w253) -> ("Mean Rp"=w250:dbl, "Mean Cp"=w251:dbl)
        n118 = local read "LCR Params"() -> (w252:T4)
        n119 = Unbundle By Name(w257) -> ("Re(Z)"=→"ESR 3":dbl, "Ls"=→"Ls Chart 3":dbl)  [unwired: 1 out]
        n120 = Bundle By Name(cluster=w252, "Rp_Cal"=w250, "Cp_Cal"=w251) -> (w249:T4)
        n121 = local write "LCR Params"(w249) -> ()
      }
    }
    n122 = case "Timing control" shown="Default" w12 {
      frame Default {
        n123 = Get Date/Time In Seconds() -> (seconds since 1Jan1904=→"Start of current operation":timestamp)
      }
      frame "Idle" {
        # "Store the last start time point for all system states that are not the \"Idle\" state. For the \"Idle\" state compute the time difference to last saved time point"
        n124 = local read "Start of current operation"() -> (w16:timestamp)
        n125 = Get Date/Time In Seconds() -> (seconds since 1Jan1904=w17:timestamp)
        n126 = Subtract(x=w17, y=w16) -> (x-y=→"Duration of last non-idle state (sec)":dbl)
      }
    }
  }
  n127 = while "Event capture loop" {
    tunnel: w5 -> [w266]
    stop <- w264 stop-if-true
    n128 = event shown="[9] \"Shunt Gain Setting 3\": Value Change" {
      selector: _ -> [_ _ _ _ _ _ _ _ _ _]
      dyn-events: _ -> [_ _ _ _ _ _ _ _ _ _]
      timeout: 100 -> [_ _ _ _ _ _ _ _ _ _]
      tunnel: [FALSE TRUE _ _ _ _ _ _ _ _] -> w265
      tunnel: w266 -> [_ w269 w275 w281 w285 w287 w291 w293 _ _]
      event Timeout {
        n129 = event-data() -> ()  [unwired: 1 in, 3 out]
      }
      event "stop": Value Change {
        n130 = event-data() -> ()  [unwired: 1 in, 6 out]
        n131 = Enqueue Element(queue=w269, element="Halt") -> ()  [unwired: 2 in, 3 out]
      }
      event "Short Comp": Value Change {
        n132 = event-data() -> ()  [unwired: 1 in, 6 out]
        n133 = Enqueue Element(queue=w275, element="Update System Variables") -> (queue out=w274:refnum<queue>)  [unwired: 2 in, 2 out]
        n134 = Enqueue Element(queue=w274, element="Short Compensation") -> (queue out=w271:refnum<queue>)  [unwired: 2 in, 2 out]
        n135 = Enqueue Element(queue=w271, element="Update System Variables") -> ()  [unwired: 2 in, 3 out]
      }
      event "Open Comp": Value Change {
        n136 = event-data() -> ()  [unwired: 1 in, 6 out]
        n137 = Enqueue Element(queue=w281, element="Update System Variables") -> (queue out=w280:refnum<queue>)  [unwired: 2 in, 2 out]
        n138 = Enqueue Element(queue=w280, element="Open Compensation") -> (queue out=w277:refnum<queue>)  [unwired: 2 in, 2 out]
        n139 = Enqueue Element(queue=w277, element="Update System Variables") -> ()  [unwired: 2 in, 3 out]
      }
      event "Start Stats": Value Change {
        n140 = event-data() -> ()  [unwired: 1 in, 6 out]
        n141 = Enqueue Element(queue=w285, element="Update System Variables") -> (queue out=w284:refnum<queue>)  [unwired: 2 in, 2 out]
        n142 = Enqueue Element(queue=w284, element="Measure Impedance Stats") -> ()  [unwired: 2 in, 3 out]
      }
      event "Update Variables": Value Change {
        n143 = event-data() -> ()  [unwired: 1 in, 6 out]
        n144 = Enqueue Element(queue=w287, element="Update System Variables") -> ()  [unwired: 2 in, 3 out]
      }
      event "Start Freq. Sweep": Value Change {
        n145 = event-data() -> ()  [unwired: 1 in, 6 out]
        n146 = Enqueue Element(queue=w291, element="Update System Variables") -> (queue out=w289:refnum<queue>)  [unwired: 2 in, 2 out]
        n147 = Enqueue Element(queue=w289, element="Freq. Sweep") -> ()  [unwired: 2 in, 3 out]
      }
      event "Start Single Meas": Value Change {
        n148 = event-data() -> ()  [unwired: 1 in, 6 out]
        n149 = Enqueue Element(queue=w293, element="Update System Variables") -> (queue out=w294:refnum<queue>)  [unwired: 2 in, 2 out]
        n150 = Enqueue Element(queue=w294, element="Single Meas") -> ()  [unwired: 2 in, 3 out]
      }
      event "Shunt Gain Setting": Value Change {
        n151 = event-data() -> ()  [unwired: 1 in, 6 out]
        n152 = call "SetResetRelay.vi"("SetLine"="SetLine-Shunt", "ResetLine"="ResetLine-Shunt", "Set=T,Rst=F"="Shunt Gain Setting") -> ()  [unwired: 9 in]
        n153 = local read "LCR Params"() -> (w302:T4)
        n154 = Select(t=10000.0, s="Shunt Gain Setting", f=499.0) -> (s? t:f=w298:dbl)
        n155 = Bundle By Name(cluster=w302, "R_Shunt"=w298) -> (w297:T4)
        n156 = local write "LCR Params"(w297) -> ()
      }
      event "Shunt Gain Setting 3": Value Change {
        n157 = event-data() -> ()  [unwired: 1 in, 6 out]
        n158 = call "SetResetRelay.vi"("SetLine"="SetLine-Shunt 2", "ResetLine"="ResetLine-Shunt 2", "Set=T,Rst=F"="Shunt Gain Setting 3") -> ()  [unwired: 9 in]
      }
    }
    n159 = local read "Main loop has stopped"() -> (w263:bool)
    n160 = Or(x=w265, y=w263) -> (x .or. y?=w264:bool)
  }
  n161 = local write "Main loop has stopped"(w1) -> ()
  "Main loop has stopped" <- FALSE ("Main loop has stopped")
